vi "sanitize.vi"(11 "Input":i32) -> (3 "Sanitized Input":i32)   [LabVIEW 2019]
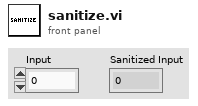
[diagram p1: front panel]
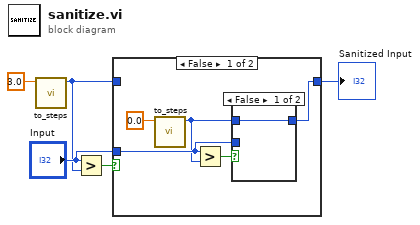
[diagram p0: block diagram]
diagram:
  n1 = call "to_steps.vi"("Turns"=3.0) -> ("Steps"=w2:i32)  [unwired: 10 in]
  n2 = Greater?(x="Input", y=w2) -> (0:w5:bool)
  n3 = case shown="False" w5 {
    tunnel: [w9 w13] -> w4
    tunnel: w2 -> [_ w13]
    tunnel: "Input" -> [w8 _]
    frame False {
      n4 = call "to_steps.vi"("Turns"=0.0) -> ("Steps"=w7:i32)  [unwired: 10 in]
      n5 = Greater?(x=w8, y=w7) -> (0:w10:bool)
      n6 = case shown="False" w10 {
        tunnel: [w11 w12] -> w9
        tunnel: w8 -> [_ w12]
        tunnel: w7 -> [w11 _]
        frame False {
        }
        frame True {
        }
      }
    }
    frame True {
    }
  }
  "Sanitized Input" <- w4
